vi "scan & monitor2.vi"() -> ()   [LabVIEW 2011]
panel:
  in  "Boolean":bool
  out "Waveform Graph":sgl[](graph)
  out "Array":sgl[](array[numeric])
  in  "Ending Position (mm)":sgl
  in  "Starting Position (mm)":sgl
  in  "HWSerialNum":i32=83837638
  in  "MG17Motor":refnum<k7>(container)
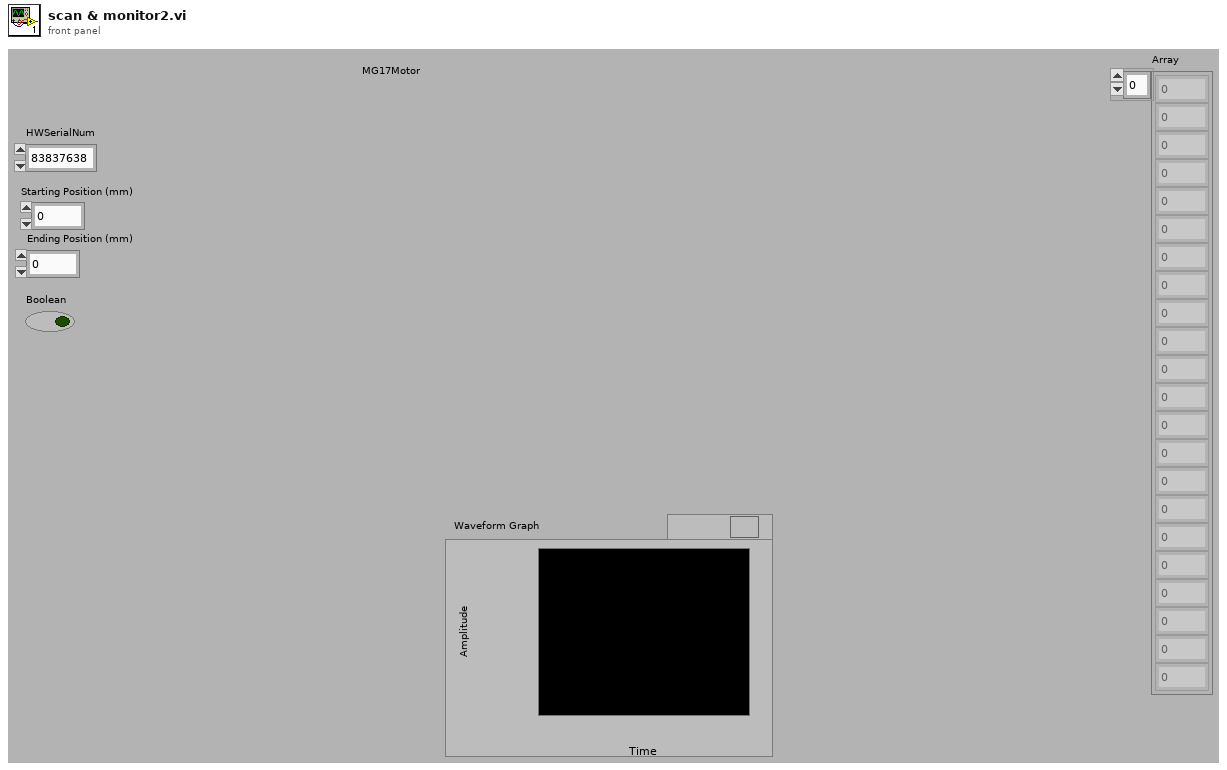
[diagram p1: front panel]
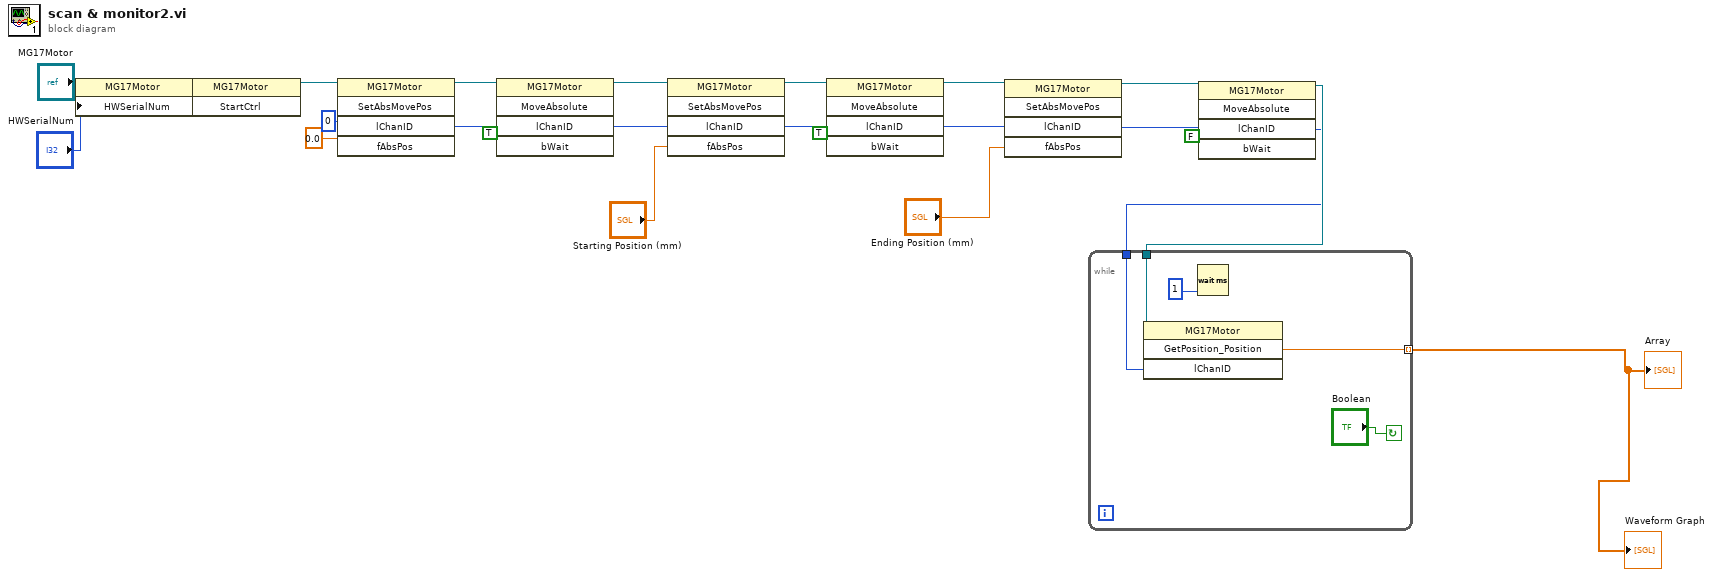
[diagram p0: block diagram]
diagram:
  n1 = property class="MG17Motor"(reference="MG17Motor", "HWSerialNum"="HWSerialNum") -> (reference out=w22:refnum<k7>)  [unwired: 1 in, 1 out]
  n2 = invoke class="MG17Motor" method="StartCtrl"(reference=w22) -> (reference out=w5:refnum<k7>)  [unwired: 2 in, 2 out]
  n3 = invoke class="MG17Motor" method="SetAbsMovePos"(reference=w5, "lChanID"=0, "fAbsPos"=sgl 0.0) -> (reference out=w7:refnum<k7>, "lChanID"=w8:i32)  [unwired: 2 in, 3 out]
  n4 = invoke class="MG17Motor" method="MoveAbsolute"(reference=w7, "lChanID"=w8, "bWait"=TRUE) -> (reference out=w3:refnum<k7>, "lChanID"=w4:i32)  [unwired: 2 in, 3 out]
  n5 = invoke class="MG17Motor" method="SetAbsMovePos"(reference=w3, "lChanID"=w4, "fAbsPos"="Starting Position (mm)") -> (reference out=w13:refnum<k7>, "lChanID"=w14:i32)  [unwired: 2 in, 3 out]
  n6 = invoke class="MG17Motor" method="MoveAbsolute"(reference=w13, "lChanID"=w14, "bWait"=TRUE) -> (reference out=w20:refnum<k7>, "lChanID"=w15:i32)  [unwired: 2 in, 3 out]
  n7 = invoke class="MG17Motor" method="SetAbsMovePos"(reference=w20, "lChanID"=w15, "fAbsPos"="Ending Position (mm)") -> (reference out=w12:refnum<k7>, "lChanID"=w11:i32)  [unwired: 2 in, 3 out]
  n8 = invoke class="MG17Motor" method="MoveAbsolute"(reference=w12, "lChanID"=w11, "bWait"=FALSE) -> (reference out=w2:refnum<k7>, "lChanID"=w1:i32)  [unwired: 2 in, 3 out]
  n9 = while {
    tunnel: [w28] -> w17 mode=indexing
    tunnel: w2 -> [w26]
    tunnel: w1 -> [w25]
    stop <- "Boolean" continue-if-true
    n10 = invoke class="MG17Motor" method="GetPosition_Position"(reference=w26, "lChanID"=w25) -> ("GetPosition_Position"=w28:sgl)  [unwired: 2 in, 3 out]
    n11 = Wait (ms)(milliseconds to wait=u32 1) -> ()  [unwired: 1 out]
  }
  "Array" <- w17
  "Waveform Graph" <- w17
